vi "Write Sample Transfer.Sample In Transfer.vi"(10 "Sample.lvclass":refnum<class "Sample.lvclass">, 11 "cRIO-CO2 in":refnum<class "cRIO-CO2.lvclass">) -> (3 "cRIO-CO2 out":refnum<class "cRIO-CO2.lvclass">)   [LabVIEW 2015, in "cRIO-Carbondioxide.lvlib" / "cRIO-CO2.lvlib" / "cRIO-CO2.lvclass"]
uses:
  cRIO-CO2.lvclass
  subs/Sample/Sample.lvclass
  cRIO-CO2.lvclass/cRIO-CO2.ctl
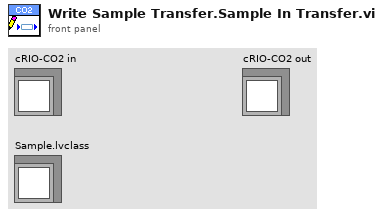
[diagram p1: front panel]
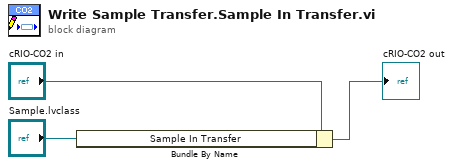
[diagram p0: block diagram]
diagram:
  n1 = Bundle By Name(cluster="cRIO-CO2 in", "Sample In Transfer"="Sample.lvclass") -> (→"cRIO-CO2 out":refnum<class "cRIO-CO2.lvclass">)
